vi "MCL Move Z Center.vi"(9 "handle":i32, 10 "actual":dbl, 11 "position":dbl) -> (2 "actual out":dbl, 3 "function return":i32)   [LabVIEW 2017, in "Madlib.lvlib"]
doc: "MADLIB_API int MCL_MoveZCenter(double position, double *actual, int handle);"
uses:
  Madlib.lvlib
  Madlib.dll
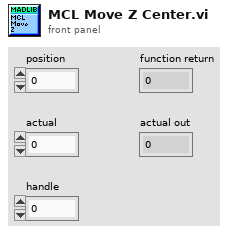
[diagram p1: front panel]
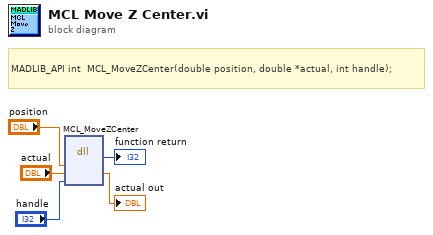
[diagram p0: block diagram]
diagram:
  # "MADLIB_API\tint\t\tMCL_MoveZCenter(double position, double *actual, int handle);"
  n1 = dll-call lib="C:/Users/francesco/dev/pump-probe/Piezo/lvlib/Madlib.*" fn="MCL_MoveZCenter"("position"="position", "actual"="actual", "handle"="handle") -> (→"function return":i32, "actual"=→"actual out":dbl)  [unwired: 5 in, 2 out]
